vi "channeldata_continued_interleaved.vi"() -> ()   [LabVIEW 2019]
panel:
  out "Error Out":errorcluster
  in  "TDMS File":path=path "C:/Python/projects/nitdms/tests/tdms_files/channeldata_continued_interleaved.tdms"
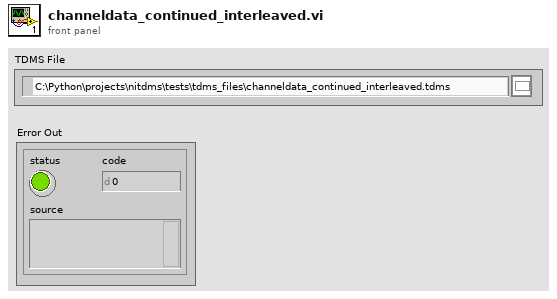
[diagram p1: front panel]
types:
  T1 = enum16{"open", "open or create", "create or replace", "create", "open (read-only)"}
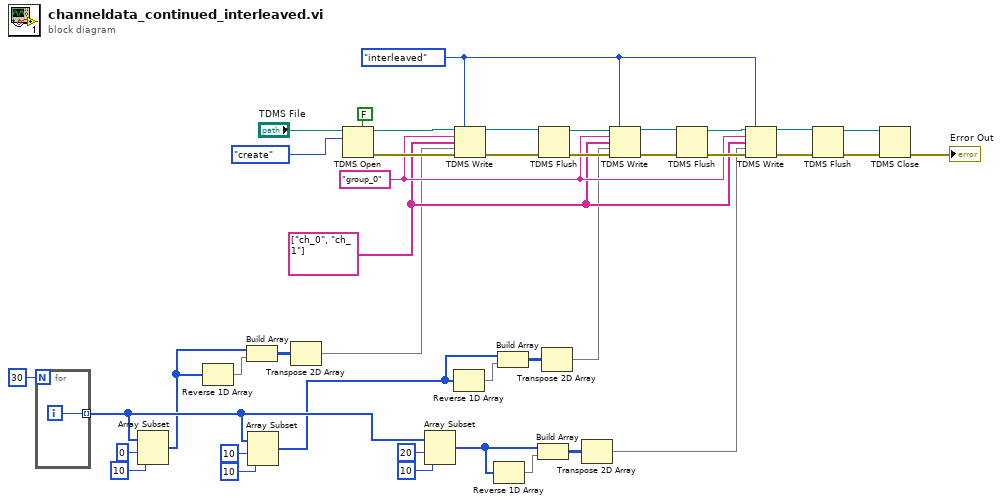
[diagram p0: block diagram]
diagram:
  w13 = enum16{"decimated", "interleaved"}."interleaved" ("data layout (0:decimated)")
  w14 = string[] ["ch_0", "ch_1"]
  w15 = "group_0"
  n1 = for {
    N: 30 -> [_]
    tunnel: [w42] -> w28 mode=indexing
    i -> [w42]
  }
  n2 = Array Subset(array=w28, index=0, length=10) -> (w11:i32[])
  n3 = Reverse 1D Array(array=w11) -> (reversed array=w12:i32[])
  n4 = Build Array(w11, w12) -> (w10:i32[][])
  n5 = Array Subset(array=w28, index=10, length=10) -> (w6:i32[])
  n6 = Transpose 2D Array(2D array=w10) -> (transposed array=w9:i32[][])
  n7 = TDMS Open(5:FALSE ("create index file? (T)"), 10:T1."create" ("operation (0:open)"), 11:"TDMS File") -> (0:w37:errorcluster, 3:w36:refnum<k34>)  [unwired: 4 in]
  n8 = Array Subset(array=w28, index=20, length=10) -> (w2:i32[])
  n9 = Reverse 1D Array(array=w6) -> (reversed array=w7:i32[])
  n10 = TDMS Write(0:w36, 1:w13, 5:w15, 7:w14, 9:w9, 11:w37) -> (4:w26:refnum<k34>, 15:w27:errorcluster)  [unwired: 2 out]
  n11 = Reverse 1D Array(array=w2) -> (reversed array=w4:i32[])
  n12 = Build Array(w6, w7) -> (w8:i32[][])
  n13 = Build Array(w2, w4) -> (w3:i32[][])
  n14 = TDMS Flush(4:w27, 7:w26) -> (0:w23:errorcluster, 3:w22:refnum<k34>)
  n15 = Transpose 2D Array(2D array=w8) -> (transposed array=w5:i32[][])
  n16 = Transpose 2D Array(2D array=w3) -> (transposed array=w1:i32[][])
  n17 = TDMS Write(0:w22, 1:w13, 5:w15, 7:w14, 9:w5, 11:w23) -> (4:w25:refnum<k34>, 15:w24:errorcluster)  [unwired: 2 out]
  n18 = TDMS Flush(4:w24, 7:w25) -> (0:w19:errorcluster, 3:w18:refnum<k34>)
  n19 = TDMS Write(0:w18, 1:w13, 5:w15, 7:w14, 9:w1, 11:w19) -> (4:w20:refnum<k34>, 15:w21:errorcluster)  [unwired: 2 out]
  n20 = TDMS Flush(4:w21, 7:w20) -> (0:w17:errorcluster, 3:w16:refnum<k34>)
  n21 = TDMS Close(8:w17, 11:w16) -> (0:→"Error Out":errorcluster)  [unwired: 1 out]
